vi "CallOpen.vi"(7 "Close?":bool, 8 "error in (no error)":errorcluster, 9 "DB-Name":string, 10 "Username":string, 11 "Password":string) -> (0 "error out":errorcluster, 2 "DataValid?":bool, 3 "DBref":T1)   [LabVIEW 2017, in "Server.lvlib" / "Oracle.lvlib"]
uses:
  Oracle.lvlib
  <vilib>/addons/database/Connection.llb/Conn ObjectReference.ctl
  <vilib>/addons/database/NI_Database_API.lvlib
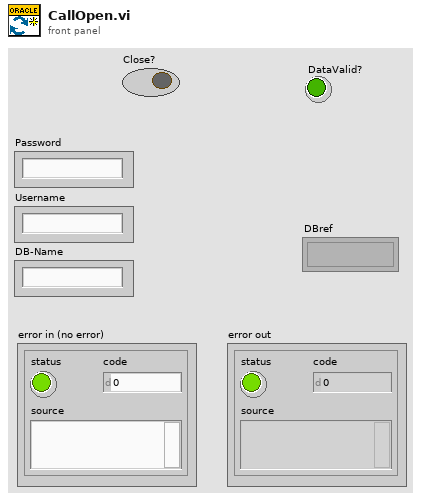
[diagram p1: front panel]
types:
  T1 = typedef "NI_Database_API.lvlib/Conn ObjectReference.ctl" = refnum<k1>
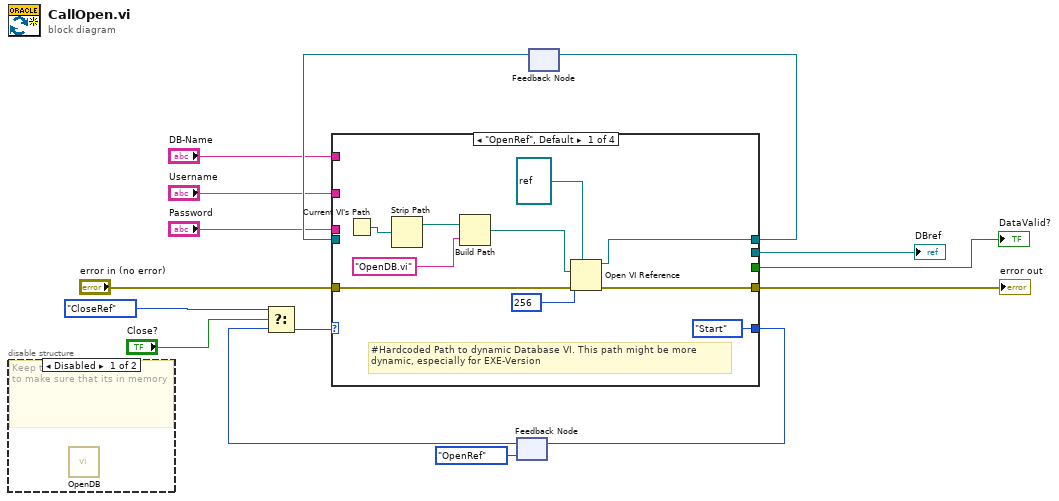
[diagram p0: block diagram]
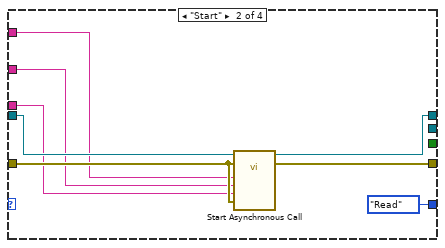
[diagram p2: hidden frame]
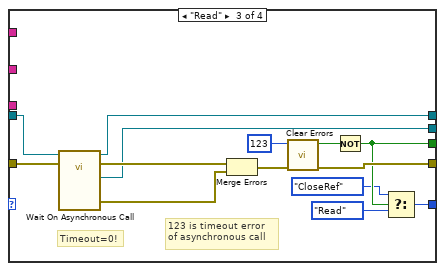
[diagram p3: hidden frame]
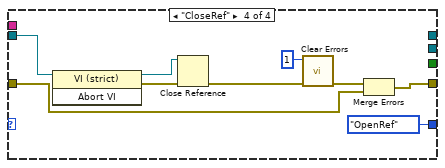
[diagram p4: hidden frame]
diagram:
  n1 = disable-structure shown="Disabled" {
    frame Disabled {
      # "Keep this VI here disabled \nto make sure that its in memory"
      n2 = call "OpenDB.vi"() -> ()  [unwired: 10 in, 2 out]
    }
    frame Enabled {
    }
  }
  n3 = feedback #1(enum16{"OpenRef", "Start", "Read", "CloseRef"}."OpenRef") -> (w11:enum16{"OpenRef", "Start", "Read", "CloseRef"})
  n4 = Select(t=enum16{"OpenRef", "Start", "Read", "CloseRef"}."CloseRef", s="Close?", f=w11) -> (s? t:f=w8:enum16{"OpenRef", "Start", "Read", "CloseRef"})
  n5 = feedback #2() -> (w10:refnum<vi>)  [unwired: 1 in]
  n6 = case shown="\"OpenRef\", Default" w8 {
    tunnel: [w24 w33 w42 w49] -> w14
    tunnel: "error in (no error)" -> [w25 w32 w47 w48]
    tunnel: [_ _ w39 _] -> w15
    tunnel: [enum16{"OpenRef", "Start", "Read", "CloseRef"}."Start" enum16{"OpenRef", "Start", "Read", "CloseRef"}."Read" w36 enum16{"OpenRef", "Start", "Read", "CloseRef"}."OpenRef" ("t")] -> w12
    tunnel: w10 -> [_ w31 w40 w54]
    tunnel: [w20 w29 w35 _] -> w5
    tunnel: [_ _ w34 _] -> w4
    tunnel: "DB-Name" -> [_ w28 _ _]
    tunnel: "Username" -> [_ w27 _ _]
    tunnel: "Password" -> [_ w26 _ _]
    frame "OpenRef", Default {
      # "#Hardcoded Path to dynamic Database VI. This path might be more\ndynamic, especially for EXE-Version"
      n7 = Current VI's Path() -> (path=w19:path)
      n8 = Strip Path(path=w19) -> (stripped path=w17:path)  [unwired: 1 out]
      n9 = Build Path(base path=w17, name or relative path="OpenDB.vi") -> (appended path=w16:path)
      n10 = Open VI Reference(type specifier VI Refnum (for type only)=refnum<vi> refnum, vi path=w16, options=256, error in (no error)=w25) -> (vi reference=w20:refnum<vi>, error out=w24:errorcluster)  [unwired: 2 in]
    }
    frame "Start" {
      n11 = call-by-ref "Start Asynchronous Call"(reference=w31, error in=w32, "Error In"=w32, "Password"=w26, "Username"=w27, "DB-Name"=w28) -> (reference out=w29:refnum<vi>, error out=w33:errorcluster)  [unwired: 6 in, 2 out]
    }
    frame "Read" {
      # "123 is timeout error\nof asynchronous call"
      # "Timeout=0!"
      n12 = call-by-ref "Wait On Asynchronous Call"(reference=w40, error in=w47) -> (reference out=w35:refnum<vi>, error out=w46:errorcluster, "Error Out"=w43:errorcluster, "DBref"=w34:T1)  [unwired: 10 in]
      n13 = Merge Errors(w46, w43) -> (w44:errorcluster)
      n14 = call <vilib>:"Clear Errors.vi"("error in (no error)"=w44, "specific error code to clear (0: all)"=123) -> ("error out"=w42:errorcluster, "specific error cleared?"=w41:bool)  [unwired: 4 in]
      n15 = Not(x=w41) -> (.not. x?=w39:bool)
      n16 = Select(t=enum16{"OpenRef", "Start", "Read", "CloseRef"}."CloseRef", s=w39, f=enum16{"OpenRef", "Start", "Read", "CloseRef"}."Read") -> (s? t:f=w36:enum16{"OpenRef", "Start", "Read", "CloseRef"})
    }
    frame "CloseRef" {
      n17 = invoke class="VI (strict)" method="Abort VI"(reference=w54) -> (reference out=w52:refnum<vi>, error out=w55:errorcluster)  [unwired: 2 in, 1 out]
      n18 = Close Reference(reference=w52, error in (no error)=w55) -> (error out=w53:errorcluster)
      n19 = call <vilib>:"Clear Errors.vi"("error in (no error)"=w53, "specific error code to clear (0: all)"=1) -> ("error out"=w51:errorcluster)  [unwired: 4 in, 1 out]
      n20 = Merge Errors(w51, w48) -> (w49:errorcluster)
    }
  }
  "DataValid?" <- w15
  "error out" <- w14
  "DBref" <- w4
  n21 = feedback-in #1(w12) -> ()
  n22 = feedback-in #2(w5) -> ()
